vi "Mod_OFDM_CAL_ERRORS.vi"(0 "Bits Received":i8[](array[numeric]), 5 "BitsTransmitted":i8[](array[numeric]), 11 "error in (no error)":errorcluster) -> (4 "O/P":T1, 15 "error out":errorcluster)   [LabVIEW 2010]
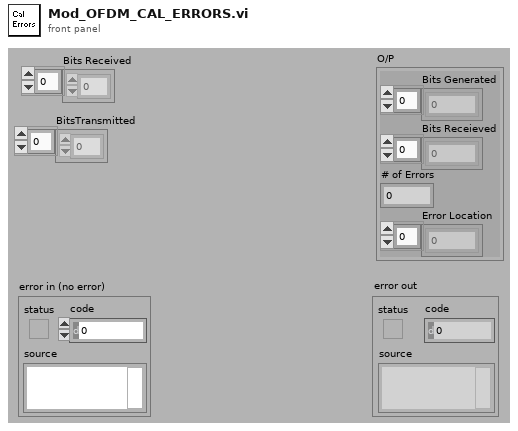
[diagram p1: front panel]
types:
  T1 = cluster{"Bits Generated":i8[], "Bits Receieved":i8[], "# of Errors":i32, "Error Location":i32[]}
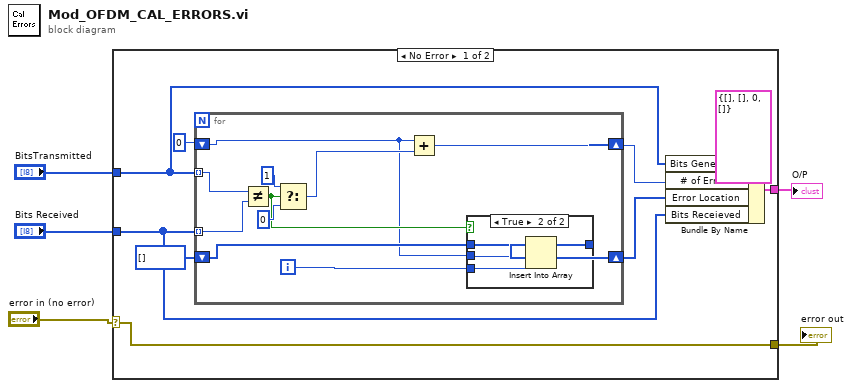
[diagram p0: block diagram]
diagram:
  n1 = case shown="No Error" "error in (no error)" {
    selector: "error in (no error)" -> [w6 w31]
    tunnel: "Bits Received" -> [w9 _]
    tunnel: "BitsTransmitted" -> [w8 _]
    tunnel: [w7 _] -> w3
    tunnel: [w6 w31] -> w1
    frame No Error {
      n2 = for {
        tunnel: w8 -> [w25] mode=indexing
        tunnel: w9 -> [w24] mode=indexing
        shift-right: [w16] -> w11
        shift-left: 0 -> [w15]
        shift-right: [w17] -> w10
        shift-left: i32[] [] -> [w18]
        i -> [w19]
        n3 = Not Equal?(x=w25, y=w24) -> (x != y?=w20:bool)
        n4 = Select(t=1, s=w20, f=0) -> (s? t:f=w21:i32)
        n5 = Add(x=w15, y=w21) -> (x+y=w16:i32)
        n6 = case shown="True" w20 {
          tunnel: w19 -> [_ w30]
          tunnel: w18 -> [w26 w29]
          tunnel: [w26 w28] -> w17
          tunnel: w15 -> [_ w27]
          frame False {
          }
          frame True {
            n7 = Insert Into Array(array=w29, index=w27, new element=w30) -> (w28:i32[])
          }
        }
      }
      n8 = Bundle By Name(cluster=T1 {"Bits Generated"=[], "Bits Receieved"=[], "# of Errors"=0, "Error Location"=[]} ("O/P"), "Bits Generated"=w8, "# of Errors"=w11, "Error Location"=w10, "Bits Receieved"=w9) -> (w7:T1)
    }
    frame Error {
    }
  }
  "O/P" <- w3
  "error out" <- w1
